vi "Print PDF.vi"(0 "Display State In":T1, 1 "printSettings":refnum<k24>, 5 "PDF File Path":path, 7 "Timeout ms":i32, 9 "Container State":T2, 11 "error in (no error)":errorcluster) -> (4 "Display State Out":T1, 6 "Timeout":bool, 15 "error out":errorcluster)   [LabVIEW 2020, in "WebView2 XControl.lvlib" / "WebView2 Control.xctl"]
uses:
  WebView2 Control.xctl
  <vilib>/_xctls/Container State.ctl
  State.ctl
  Webview2 Lib/WebView2 Control Object/WebView2 Control.lvclass
  C:/Users/Simon/Documents/GitHub/LV-WebView2/Source/Libs/Microsoft.Web.WebView2.Core.dll
  Libs/Microsoft.Web.WebView2.Core.dll
  <vilib>/_xctls/XControlSupport.lvlib
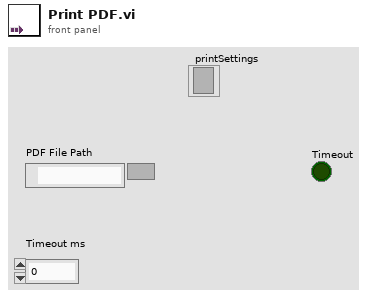
[diagram p1: front panel]
types:
  T1 = typedef "WebView2 XControl.lvlib/WebView2 Control.xctl/State.ctl" = cluster{"Control Object Ref":refnum<data-value>}
  T2 = typedef "XControlSupport.lvlib/Container State.ctl" = cluster{"Indicator?":bool, "Run Mode?":bool, " Refnum":refnum<vi>}
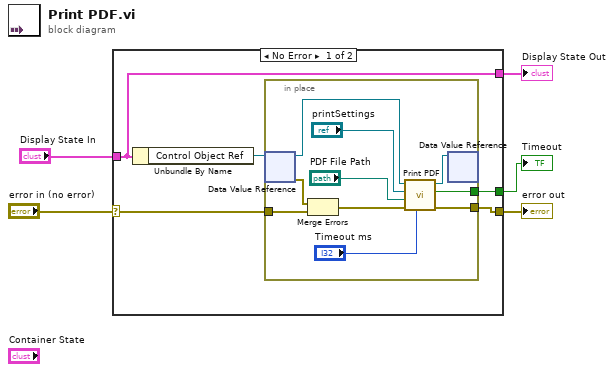
[diagram p0: block diagram]
diagram:
  n1 = case shown="No Error" "error in (no error)" {
    selector: "error in (no error)" -> [w7 w21]
    tunnel: [w8 w21] -> w5
    tunnel: [w6 _] -> w4
    tunnel: "Display State In" -> [w9 w22]
    tunnel: [w9 w22] -> w2
    frame No Error {
      n2 = Unbundle By Name(w9) -> ("Control Object Ref"=w10:refnum<data-value>)
      n3 = in-place {
        in-place-border: [w17] -> w8
        in-place-border: w7 -> [w18]
        in-place-border: [w14] -> w6
        n4 = in-place-dvr #1(w10) -> (w16:refnum<class "WebView2 Control.lvclass">, w20:errorcluster)
        n5 = Merge Errors(w20, w18) -> (w19:errorcluster)
        n6 = call "Print PDF.vi"("Timeout ms"="Timeout ms", "error in (no error)"=w19, "PDF File Path"="PDF File Path", "printSettings"="printSettings", "WebView2 Control in"=w16) -> ("error out"=w17:errorcluster, "Timeout"=w14:bool, "WebView2 Control out"=w15:refnum<class "WebView2 Control.lvclass">)  [unwired: 4 in]
        n7 = in-place-dvr #1(w15) -> ()  [unwired: 2 out]
      }
    }
    frame Error {
    }
  }
  "error out" <- w5
  "Timeout" <- w4
  "Display State Out" <- w2
